vi "cm2nm_read_session_dataFromSesionItem.vi"(2 "TopLevelDataFilePath":path, 3 "Sesions":T1) -> (1 "Session_OUT":T2)   [LabVIEW 2011]
doc: "Search logical paths for the session file. If it exists then read it and put it in Sample Set output."
uses:
  cm2nm_sample_set.ctl
  cm2nm_coordinate_information_v2.ctl
  Instrument_type_enum_v2.ctl
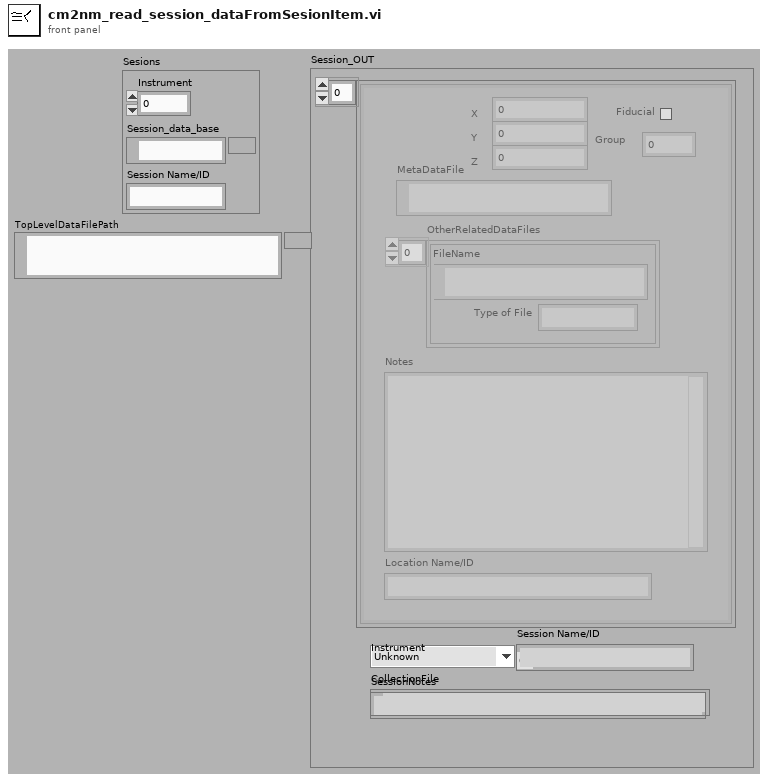
[diagram p1: front panel]
types:
  T1 = cluster{"Instrument":u16, "Session_data_base":path, "Session Name/ID":string}
  T2 = typedef "cm2nm_sample_set.ctl" = cluster{"CollectionOfPoints":T3[], "Instrument":T4, "CollectionFile":path, "Session Name/ID":string, "SessionNotes":string}
  T3 = typedef "cm2nm_coordinate_information_v2.ctl" = cluster{"MetaDataFile":path, "X":dbl, "Y":dbl, "Z":dbl, "Group":i32, "Rotation":dbl[unit], "Fiducial":bool, "Magnification":dbl, "Working_Distance":dbl, "Notes":string, "Location Name/ID":string, "OtherRelatedDataFiles":cluster{"Type of File":string, "FileName":path}[], "Available":bool}
  T4 = typedef "Instrument_type_enum_v2.ctl" = enum16{"Unknown", "Philips FEI SEM IRC", "JEOL 7000F EML_MFC", "MXRD MFC", "JEOL_EPMA"}
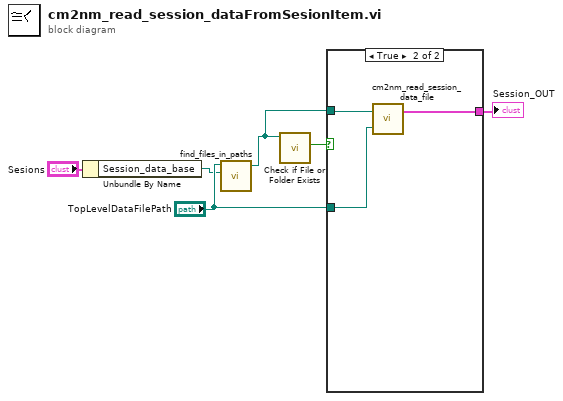
[diagram p0: block diagram]
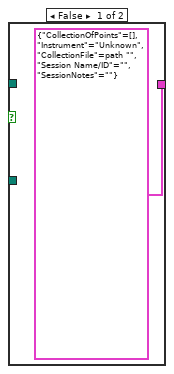
[diagram p2: hidden frame]
diagram:
  n1 = Unbundle By Name("Sesions") -> ("Session_data_base"=w2:path)
  n2 = call "find_files_in_paths.vi"("TopLevelDataFilePath"="TopLevelDataFilePath", "File2Find"=w2) -> ("Path"=w1:path)  [unwired: 4 in, 1 out]
  n3 = call <vilib>:"Check if File or Folder Exists.vi"("path"=w1) -> ("file or folder exists?"=w4:bool)  [unwired: 8 in, 2 out]
  n4 = case shown="True" w4 {
    tunnel: [T2 {"CollectionOfPoints"=[], "Instrument"=enum."Unknown", "CollectionFile"=path "", "Session Name/ID"="", "SessionNotes"=""} ("Sample Set") w10] -> w6
    tunnel: w1 -> [_ w9]
    tunnel: "TopLevelDataFilePath" -> [_ w8]
    frame False {
    }
    frame True {
      n5 = call "cm2nm_read_session_data_file.vi"("TopLevelDataFilePath"=w8, "Session_data_base"=w9) -> ("Session Information"=w10:T2)  [unwired: 1 in]
    }
  }
  "Session_OUT" <- w6
